vi "Main On Load Action VI.vi"(8 "error in (no error)":errorcluster, 11 "Device Item Ref in":T1 format="%.0x") -> (0 "error out":errorcluster, 3 "Device Item Ref out":T1 format="%.0x")   [LabVIEW 2015, in "AIT 664 Custom Device.lvlib"]
uses:
  AIT 664 Custom Device.lvlib
  <vilib>/NI Veristand/Custom Device API/Custom Device Item Ref.ctl
  <vilib>/NI Veristand/Custom Device API/Custom Device Path Data.ctl
  <vilib>/NI Veristand/Custom Device API/Custom Device Supported Target.ctl
  <vilib>/NI Veristand/Custom Device API/Path Specification.ctl
  <vilib>/NI Veristand/Custom Device API/Path Type.ctl
  <vilib>/NI Veristand/Custom Device API/Custom Device Execution Mode.ctl
  <vilib>/NI Veristand/Custom Device API/Custom Device API.lvlib
  NationalInstruments.VeriStand.SystemDefinitionAPI
  Controls and Global/Global.vi
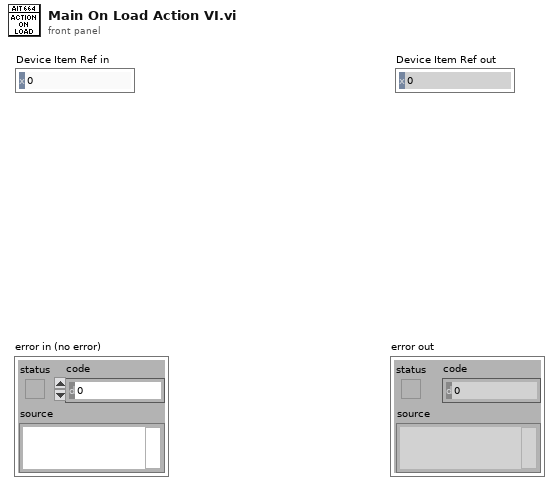
[diagram p1: front panel]
types:
  T1 = typedef "Custom Device API.lvlib/Custom Device Item Ref.ctl" = u64
  T2 = typedef "Custom Device API.lvlib/Path Specification.ctl" = cluster{"Path":path, "Type":T3}
  T3 = typedef "Custom Device API.lvlib/Path Type.ctl" = enum16{"Absolute", "To Base", "To Common Data Dir", "To Application Data Dir"}
  T4 = typedef "Custom Device API.lvlib/Custom Device Execution Mode.ctl" = enum16{"Asynchronous", "Inline HW Interface", "Inline Model Interface", "Inline Timing and Sync", "Asynchronous Timing and Sync"}
  T5 = typedef "Custom Device API.lvlib/Custom Device Supported Target.ctl" = enum16{"All", "PharLap", "VxWorks", "Windows", "Linux_32_ARM", "Linux_x64", "PharLap & Windows", "PharLap & VxWorks", "VxWorks & Windows"}
  T6 = typedef "Custom Device API.lvlib/Custom Device Path Data.ctl" = cluster{"SupportedTarget":T5, "Source":T2, "RT Destination":path}
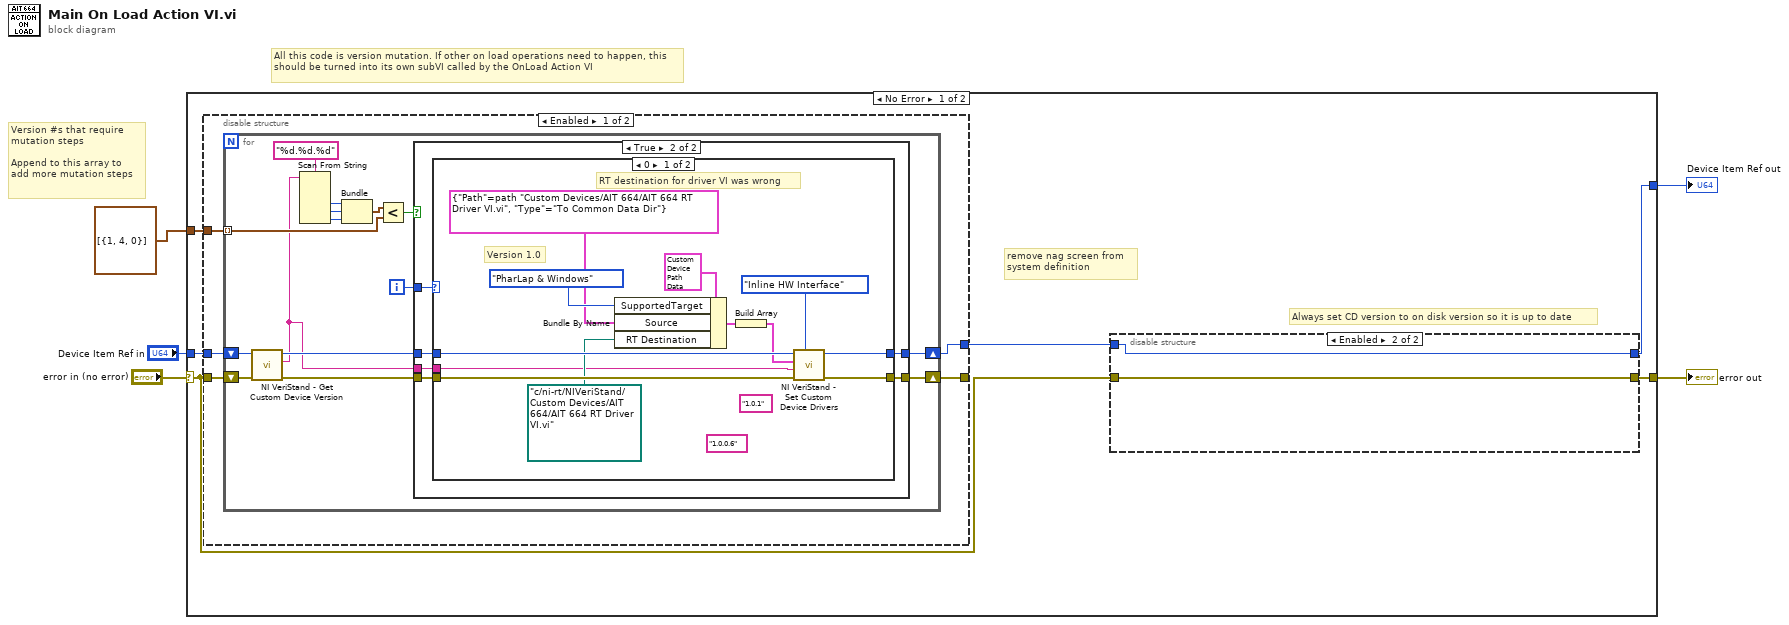
[diagram p0: block diagram]
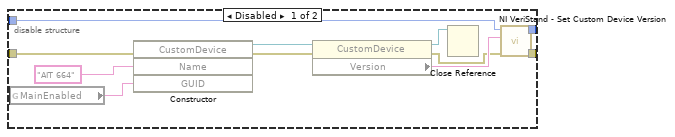
[diagram p2: hidden frame]
diagram:
  # "All this code is version mutation. If other on load operations need to happen, this should be turned into its own subVI called by the OnLoad Action VI"
  # "Version #s that require\nmutation steps\n\nAppend to this array to\nadd more mutation steps"
  n1 = case shown="No Error" "error in (no error)" {
    selector: "error in (no error)" -> [w6 w70]
    tunnel: [w9 w70] -> w4
    tunnel: "Device Item Ref in" -> [w10 w69]
    tunnel: [w8 w69] -> w2
    tunnel: cluster{i32, i32, i32}[] [{1, 4, 0}] -> [w11 _]
    frame No Error {
      # "remove nag screen from\nsystem definition"
      # "Always set CD version to on disk version so it is up to date"
      n2 = disable-structure shown="Enabled" {
        disable-tunnel: w11 -> [w29 _]
        disable-tunnel: w6 -> [w28 w67]
        disable-tunnel: w10 -> [w27 w68]
        disable-tunnel: [w26 w67] -> _
        disable-tunnel: [w25 w68] -> w7
        frame Enabled {
          n3 = for {
            tunnel: w29 -> [w32] mode=indexing
            shift-right: [w36] -> w26
            shift-left: w28 -> [w40]
            shift-right: [w34] -> w25
            shift-left: w27 -> [w39]
            i -> [w33]
            n4 = call <vilib>:"NI VeriStand - Get Custom Device Version.vi"("error in (no error)"=w40, "Device Ref in"=w39) -> ("error out"=w37:errorcluster, "Value"=w30:string, "Device Ref out"=w35:T1)  [unwired: 7 in]
            n5 = Scan From String(format string="%d.%d.%d", input string=w30) -> (output 1=w42:i32, output 2=w43:i32, output 3=w31:i32)  [unwired: 5 in, 3 out]
            n6 = Bundle(w42, w43, w31) -> (w44:cluster{i32, i32, i32})  [unwired: 1 in]
            n7 = Less?(x=w44, y=w32) -> (x < y?=w38:bool)
            n8 = case shown="True" w38 {
              tunnel: w37 -> [w46 w52]
              tunnel: [w46 w51] -> w36
              tunnel: w35 -> [w45 w48]
              tunnel: [w45 w49] -> w34
              tunnel: w33 -> [_ w50]
              tunnel: w30 -> [_ w47]
              frame False {
              }
              frame True {
                n9 = case shown="0" w50 {
                  tunnel: w52 -> [w62 w66]
                  tunnel: [w55 w66] -> w51
                  tunnel: [w64 w65] -> w49
                  tunnel: w48 -> [w61 w65]
                  tunnel: w47 -> [w53 _]
                  frame 0 {
                    (unwired) "1.0.0.6" ("format string")
                    (unwired) "1.0.1" ("format string")
                    # "RT destination for driver VI was wrong"
                    # "Version 1.0"
                    n10 = Bundle By Name(cluster=T6 {"SupportedTarget"=enum."All", "Source"={"Path"=path "", "Type"=enum."Absolute"}, "RT Destination"=path ""} ("Driver VI Path"), "SupportedTarget"=Custom_Device_Supported_Target."PharLap & Windows", "Source"=T2 {"Path"=path "Custom Devices/AIT 664/AIT 664 RT Driver VI.vi", "Type"=enum."To Common Data Dir"}, "RT Destination"=path "c:/ni-rt/NIVeriStand/Custom Devices/AIT 664/AIT 664 RT Driver VI.vi") -> (w59:T6)
                    n11 = Build Array(w59) -> (w58:T6[])
                    n12 = call <vilib>:"NI VeriStand - Set Custom Device Drivers.vi"("Execution mode"=Custom_Device_Execution_Mode."Inline HW Interface", "error in (no error)"=w62, "Version"=w53, "Driver VI"=w58, "Device Ref in"=w61) -> ("error out"=w55:errorcluster, "Device Ref out"=w64:T1)  [unwired: 5 in]
                  }
                  frame Default {
                  }
                }
              }
            }
          }
        }
        frame Disabled {
        }
      }
      n13 = disable-structure shown="Enabled" {
        disable-tunnel: [w17 w23] -> w9
        disable-tunnel: [w16 w24] -> w8
        disable-tunnel: w7 -> [w14 w24]
        disable-tunnel: w6 -> [w13 w23]
        frame Disabled {
          n14 = global read "Global.vi" "MainEnabled"() -> (w15:string)
          n15 = constructor class="CustomDevice"(error in=w13, "Name"="AIT 664", "GUID"=w15) -> (reference out=w21:refnum<k24>, error out=w20:errorcluster)  [unwired: 2 in, 3 out]
          n16 = property class="CustomDevice"(reference=w21, error in=w20) -> (reference out=w19:refnum<k24>, error out=w12:errorcluster, "Version"=w18:string)
          n17 = Close Reference(reference=w19) -> ()  [unwired: 1 in, 1 out]
          n18 = call <vilib>:"NI VeriStand - Set Custom Device Version.vi"("error in (no error)"=w12, "Value"=w18, "Device Ref in"=w14) -> ("error out"=w17:errorcluster, "Device Ref out"=w16:T1)  [unwired: 7 in]
        }
        frame Enabled {
        }
      }
    }
    frame Error {
    }
  }
  "error out" <- w4
  "Device Item Ref out" <- w2
